vi "HydroCal.vi"() -> ()   [LabVIEW 2022 SP3]
uses:
  ScanningControl/Motion Controllers/NI_controller/-NI_MotionRoutines/MotionSys.ctl
  ScanningControl/Motion Controllers/-MotionRoutines/ScanAxis.ctl
  <vilib>/Math Plots/3D Math Plots/3D Surface/3D Surface XCtrl/3D Surface.xctl
  -CalTransducer/HydrophoneSettings.ctl
  -CalTransducer/Hydros.ctl
  ScanningControl/Digitizers/-DigitizerRoutines/DigitizerSettings.ctl
  ScanningControl/Digitizers/-DigitizerRoutines/Digitizer.ctl
  ScanningControl/Digitizers/-DigitizerRoutines/DigConfig.ctl
  ScanningControl/Digitizers/-DigitizerRoutines/DigitizerID.ctl
  <instrlib>/niSwitch/niSwitch.llb/niSwitch Topologies.ctl
  ScanningControl/Motion Controllers/NI_controller/-NI_MotionRoutines/MotionParameters.ctl
  ScanningControl/Motion Controllers/-MotionRoutines/3rdAxis.ctl
  <vilib>/Analysis/baseanly.llb/Mean (DBL).vi
  <vilib>/Analysis/5stat.llb/RMS (DBL).vi
  ScanningControl/Motion Controllers/-MotionRoutines/MotionGlobals.vi
  <instrlib>/niSwitch/niSwitch.llb/niSwitch Connect Channels (Single).vi
  <vilib>/Math Plots/3D Math Plots/3D Surface/3D Surface Datatype/Public/Plot Helper (Vector).vi
  <instrlib>/niScope/Acquire/Fetch/niScope Multi Fetch.vi
  <vilib>/Utility/file.llb/Write To Spreadsheet File (DBL).vi
  C:/Windows/System32/ADQAPI_dotNet_helper.dll
  <vilib>/Analysis/NI_AALPro.lvlib
  <vilib>/Math Plots/3D Math Plots/3D Surface/3D Surface Datatype/3D Surface Datatype.lvclass
  <vilib>/Analysis/NI_AALBase.lvlib
panel:
  in  "Pressure Cal Parameters":T1={"Center Freq (MHz)"=0.0, "PRF (kHz)"=1.0, "Pulse window (us)"=0.0, "Hydrophone"=enum."PAL #1048", "booster amp?"=TRUE} {"Pulse window (us)" format="%.2f"; "PRF (kHz)" format="%.2f"; "Center Freq (MHz)" format="%.2f"}
  in  "data out":dbl[][][](array[numeric])
  in  "reset mux":bool=TRUE caption="reset mx"
  in  "FileName":string="H"
  in  "Folder":path=path "E:/Temp"
  out "Current Element":i32
  in  "Plot":enum32{"1-D", "2-D", "data", "Spectra"}(tab)
  out "XY Graph":cluster{"axis 1 ticks":dbl[], "data out":dbl[]}(graph)
  in  "Scan":i16=20
  out "3D Surface":refnum<class "3D Plot Datatype.lvclass">[](xcontrol)
  out "Raw Waveforms":dbl[][](graph)
  out "Rms":dbl[](graph)
  out "centers":dbl[][](array[numeric])
  out "Waveform Graph":cluster{i32, "df":dbl, dbl[][]}(graph)
  in  "FFT size":u16(ring) items=["next 2^n", "8", "16", "32", "64", "128", "256", "512", "1024", "2056"]
  in  "home":bool
  in  "Man Cont":bool
  in  "Set up Digi":bool
  in  "Element spacing (mm)":dbl=-1.25
  in  "Elements":i16=20
  in  "scan pair":T3
  in  "Motion System":T4=enum."No Motion Card"
  in  "Motion Bd ID":u8=1 min=1 max=32 step=1
  in  "Location":u16(ring) items=["RRI", "Hawaii", "Cornell", "MM Test"]
  in  "booster amp?":bool=TRUE
  out "Error Message":string
  in  "Type of scan":u16(ring) items=["1-D Scan", "2-D Scan"]
  in  "# of pts per scan":i32=11
  in  "Scan Length (mm)":dbl=5.0 format="%.2f"
  in  "scan":bool
  in  "ExitSendCmd":bool
  # "Use 2.25 unfocused Panametrics at about 65 mm standoff. 25 cycles and 100 mV from Agilent seems good. 600 rf pts seems good and offset to show start of burst. RMS values computed with 400 pts"
  # "Motion Control"
  # "© 2000-2009 WCM"
  # "Note that channels 17-20 have voltage reduced by factor of 1.0476 to account for different cable path lengths. All channels use Miteq amps."
  # "y mm"
  # "z mm"
  # "rms"
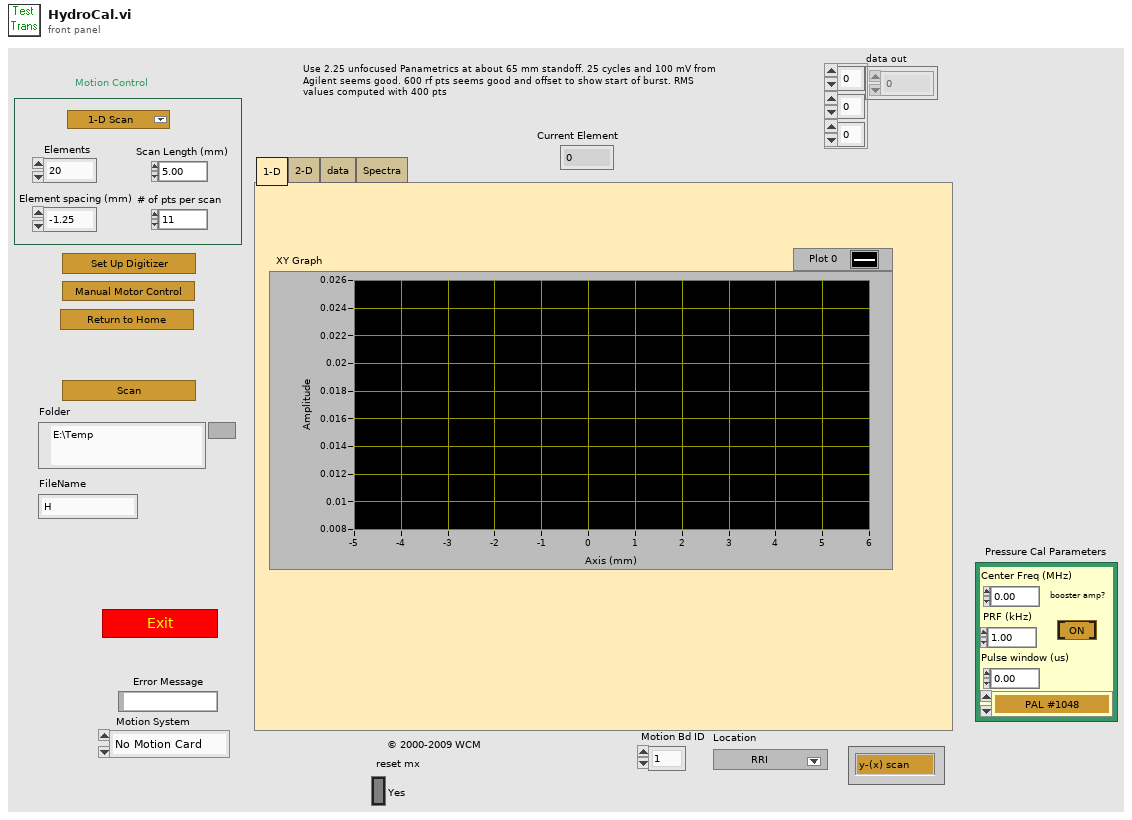
[diagram p1: front panel]
types:
  T1 = typedef "HydrophoneSettings.ctl" = cluster{"Center Freq (MHz)":dbl, "PRF (kHz)":dbl, "Pulse window (us)":dbl, "Hydrophone":T2, "booster amp?":bool}
  T2 = typedef "Hydros.ctl" = enum16{"PAL #1048", "PAL #525", "PAL #430a", "PAL #192", "DEAD PAL # 1403", "LOST UHI Onda", "DEAD PAL #1818", "PAL #1974", "DEAD #2266 w/booster", "PAL #2524 w/booster", "PAL FP21-20T", "PAL FP160-13  ", "PAL FP141-20", "PAL FP158-08T"}
  T3 = typedef "ScanAxis.ctl" = enum16{"y-(x) scan", "x-(y) scan", "z-(x) scan", "z-(y) scan", "y-(z) scan", "x-(z) scan", "w-(x) scan", "w-(y) scan", "w-(z) scan", "x-(w) scan", "y-(w) scan", "z-(w) scan"}
  T4 = typedef "MotionSys.ctl" = enum16{"MM3000", "NI 735x", "Newport ESP", "No Motion Card", "Galil"}
  T5 = typedef "DigitizerSettings.ctl" = cluster{"Digitizer delay (us) ":dbl, "rf points per line":i32, "lines per plane":i32, "Samp Rate (Hz)":dbl, "Additional dig delay (us)":dbl, "Voltage Scale":dbl, "Pre-Looks":i32, "Offset delay (us)":dbl, "bits A/D":i8, "Avg Num":i32, "DigTimeOut":sgl, "Rel Dig Delay":sgl, "Dig Ch":i32, "LeCroyCluster":cluster{"LeCroy Channels":bool[], "LC read pt offset":dbl, "Sweep Avg":bool}, "Main Digitizer":T6, "Dig Config":T7, "Digitizer ID Cluster":T8, "Trigger Settings":cluster{"Trig Source":u16, "Trig Coupling":u16, "Trig Slope":u16, "Level (mV)":dbl}, "Bulk Acq":bool, "Bulk Start Indexes":i32[], "Data Ref RF":refnum<data-value>, "NI ID/Channel":cluster{"NI ID":refnum<k15>, "NI CH":i32}[], "Total Dig CH":i32, "Xtra Ann Trig delay (us)":dbl, "Fix Z Delay?":bool, "One Way Transmission?":bool, "Data Ref Log":refnum<data-value>}
  T6 = typedef "Digitizer.ctl" = enum16{"Acqiris Digitizer", "NI Digitizer", "LeCroy", "GaGe", "AlazarTech", "No Digitizer", "Teledyne"}
  T7 = typedef "DigConfig.ctl" = enum16{"Single channel", "2 Chans w/ 2 Acqiris", "2 Chans w/ 1 Acqiris", "5-CH Pulser New", "5-CH pulser w/ ann array", "5-pass style ann array", "Empty"}
  T8 = typedef "DigitizerID.ctl" = cluster{"Acqiris/Alazar/SP ID":u32[], "NI Instr Handles":refnum<k15>[], "LeCroy VISA":refnum<visa-resource-name>, "GaGe Handle":cluster{"Handle":u32, "Sample size":u32, "Resolution":i32, "Offset":i32, "Channels":u32, "Boards":u32}, "ATS Ref":string, "Acqiris Address":string[], "ADQRef":refnum<k24>, "adq_cu_ptr":refnum<k24>}
  T9 = typedef "niSwitch Topologies.ctl" = string
  T10 = enum16{"Absolute Position", "Relative Position", "Velocity", "Relative to Cap Pos", "Modulus Position", "Absolute Contouring", "Relative Contouring"}
  T11 = typedef "MotionParameters.ctl" = cluster{"No Motion?":bool, "Motion System":T4, "Motion Bd ID":u8, "Motion Profile":string, "# Axis":i8, "Reverse Z axis?":bool, "SMAC Axis":u16, "scan pair":T3, "RT fps":sgl, "Steps per mm":i32[], "Motor Parameters":cluster{"velocity ct/s":dbl[], "accel ct/s^2":dbl[]}, "One Way Scan":bool, "Reverse One Way Scan":bool, "Global Position (mm)":dbl[], "Plane":i32, "Distance between\nscan lines (um)":sgl, "Distance between\nscan planes (um)":sgl, "number of scan planes":i32, "Total steps in line":i32, "Xtra plane\ndistance  (um)":i32, "Xtra planes ":i32, "Add Axis":bool, "overshoot cts":i32, "BKPT Shift":i32, "Scan Start Time (ms)":u32, "ESP VISA":refnum<visa-resource-name>, "3rd Axis":T12, "GL Ref Out":refnum<k7>, "Galil Address":string}
  T12 = typedef "3rdAxis.ctl" = u16
  T13 = cluster{"scan data":dbl[][][], "Pulse Parameters":cluster{"Frequency (MHz)":dbl, "prf":dbl, "focal length (cm)":dbl, "derating (.3) factor":dbl, "neg peak pressure (MPa)":dbl, "pos peak pressure (MPa)":dbl, "p.3":dbl, "pulse dur (Pd s)":dbl, "Pulse Int \nIntegral (PII J/cm^2)":dbl, "Pulse Av Intensity\n (Ipa W/cm^2)":dbl, "Ipa.3":dbl, "Temporal Av Intensity \n(Ita mW/cm^2)":dbl, "Ita.3":dbl, "MI":dbl}[][], "axis1o":dbl, "axis2o":dbl, "step size":dbl, "axis 1 ticks":dbl[], "axis 2 ticks":dbl[]}
  T14 = cluster{"actualSamples":i32, "absoluteInitialX":dbl, "relativeInitialX":dbl, "xIncrement":dbl, "offset":dbl, "gain":dbl, "reserved1":dbl, "reserved2":dbl}[]
  T15 = cluster{"actualSamples":i32, "absoluteInitialX":dbl, "relativeInitialX":dbl, "xIncrement":dbl, "offset":dbl, "gain":dbl, "reserved1":dbl, "reserved2":dbl}
  T16 = typedef "AnnularArray.ctl" = cluster{"Synth Foc?":bool, "Focal Zones":i16, "Switch T/R":i16, "Trans Geometry (mm)":T17, "Sub Ap Excite?":bool, "Full Array Scan?":bool, "Xmt/Rcv":cluster{"XMIT":bool[], "RCV":bool[]}, "PulseSpacing (us)":sgl, "Xmit Ring":i32, "XMIT CHS":u8, "RCV CHS":u8, "GPU?":bool, "Save TIFF?":bool, "downfactor":i32, "RCV 1CH":u16}
  T17 = typedef "TransGeometry.ctl" = cluster{"Transducer":T18, "Geo Focus":dbl, "a (radius)":dbl, "# of rings":i32, "kerf space ":dbl, "Center Freq":dbl}
  T18 = typedef "ArrayGeometry.ctl" = u16
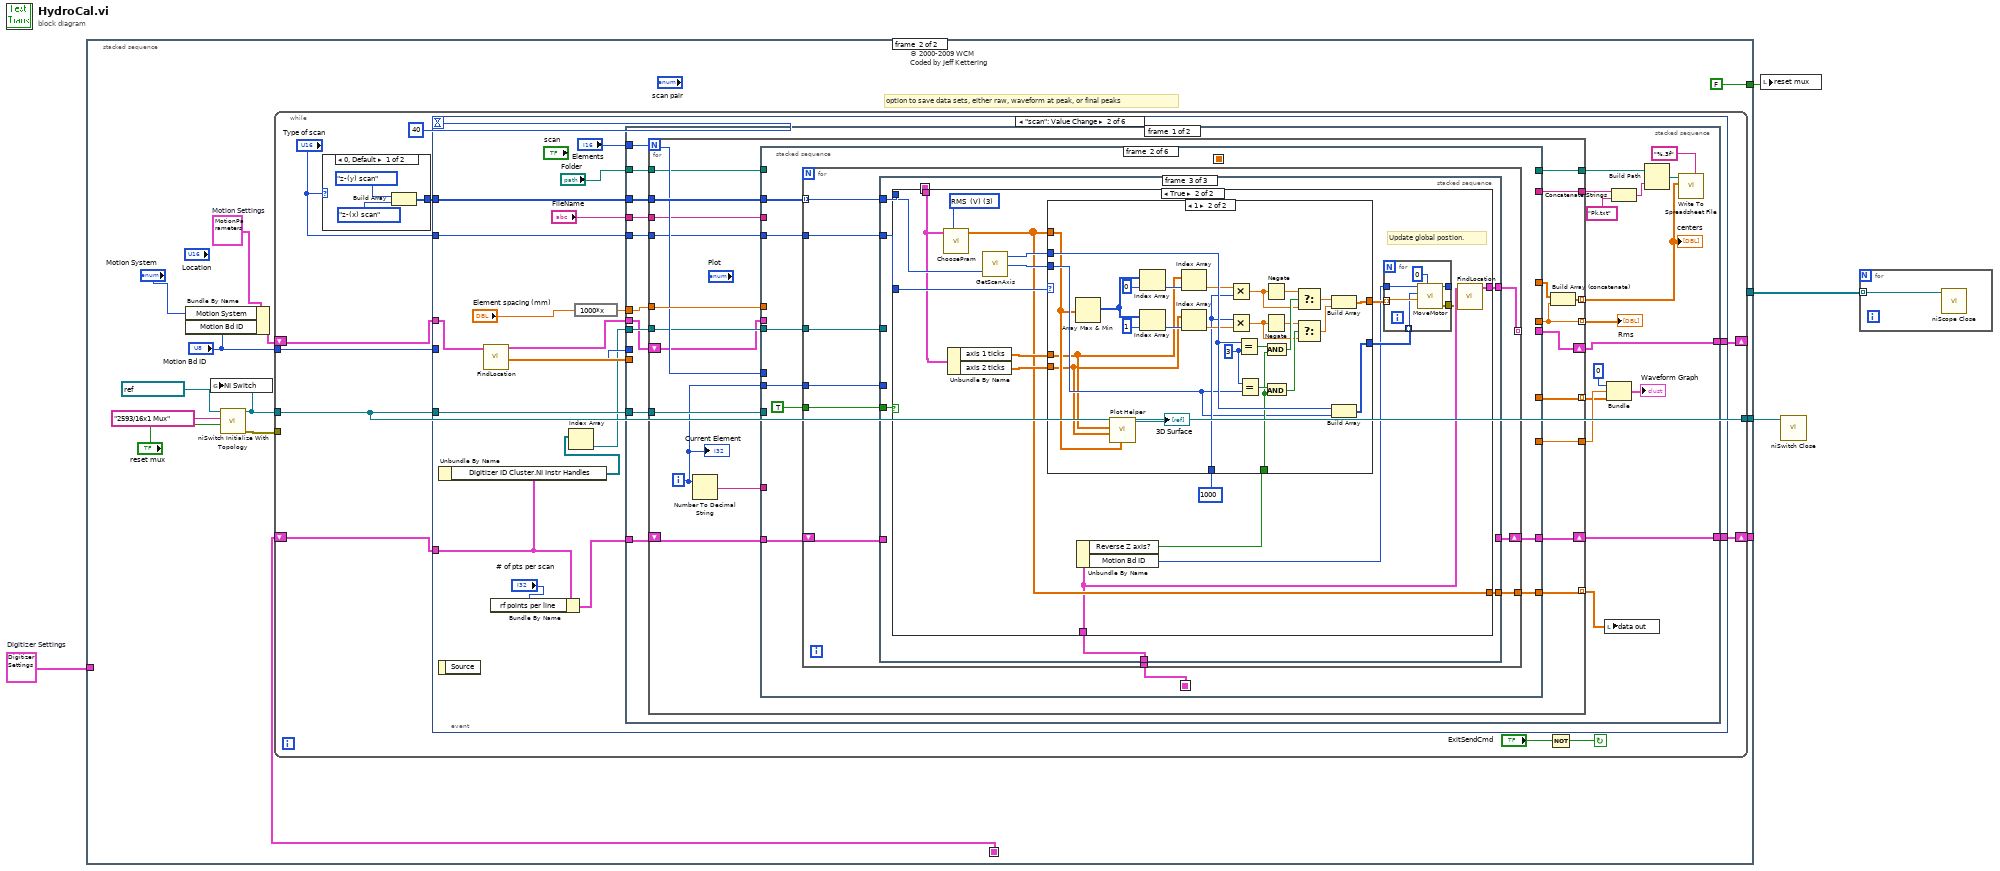
[diagram p0: block diagram]
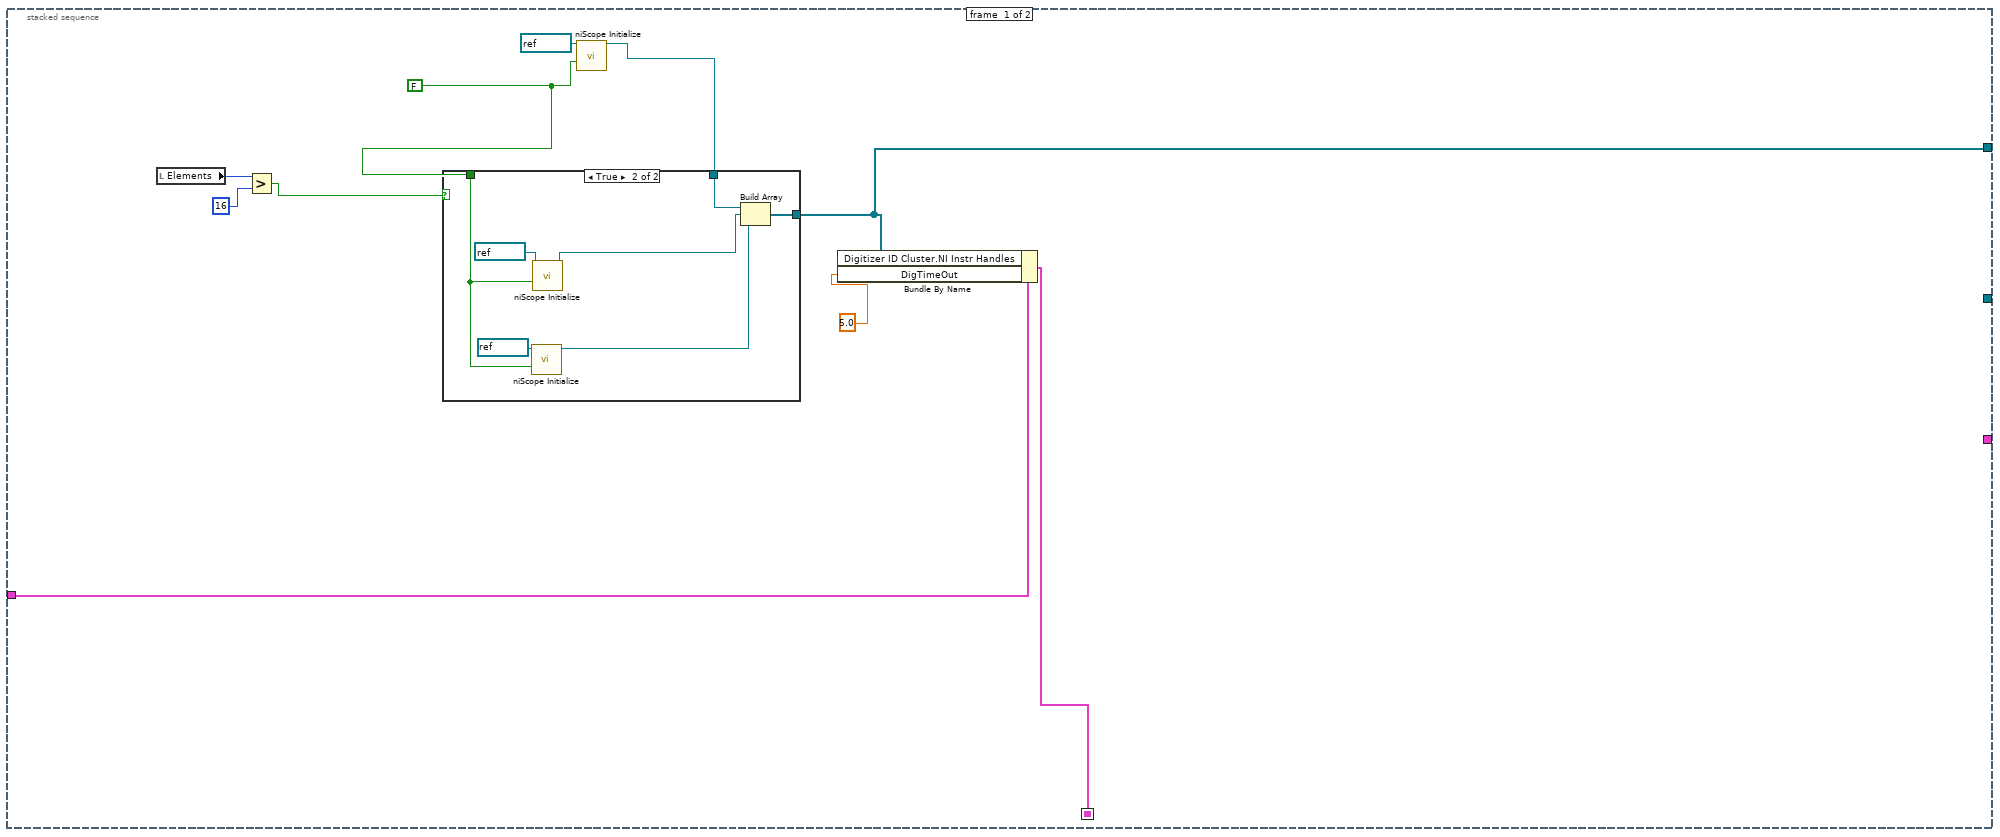
[diagram p2: hidden frame]
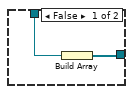
[diagram p3: hidden frame]
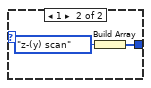
[diagram p4: hidden frame]
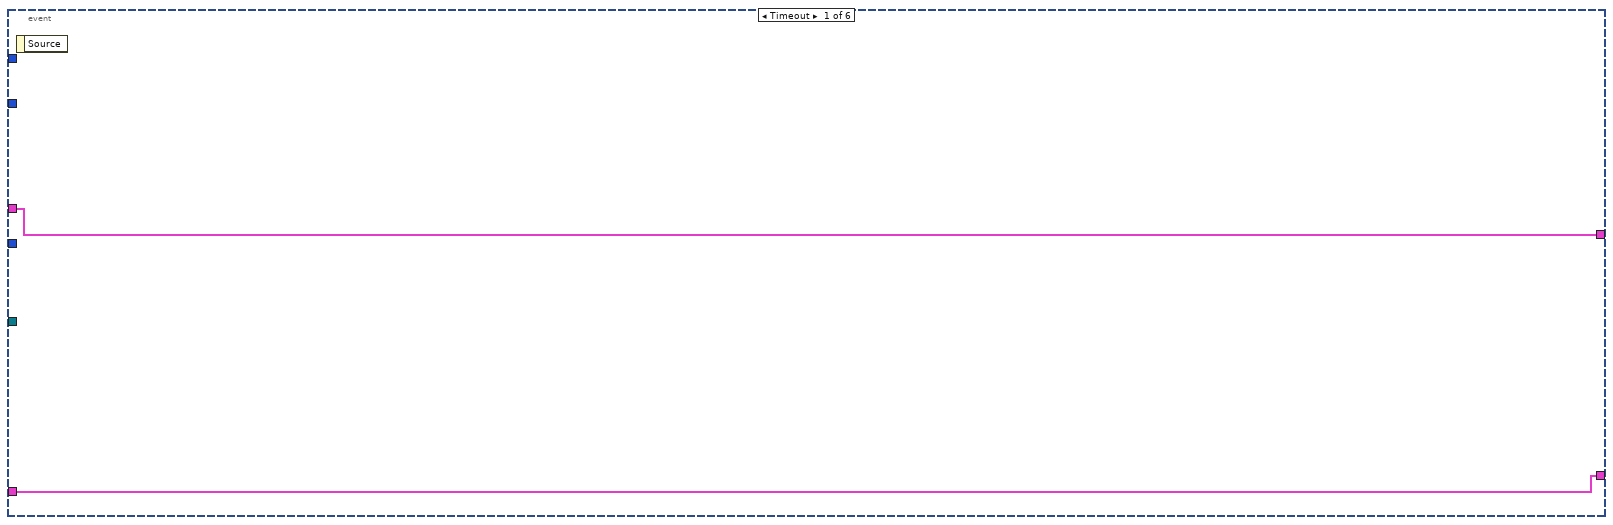
[diagram p5: hidden frame]
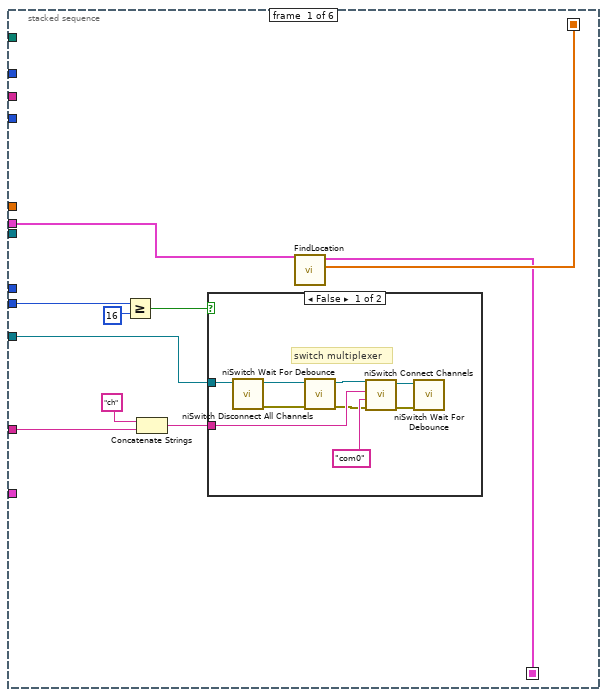
[diagram p6: hidden frame]
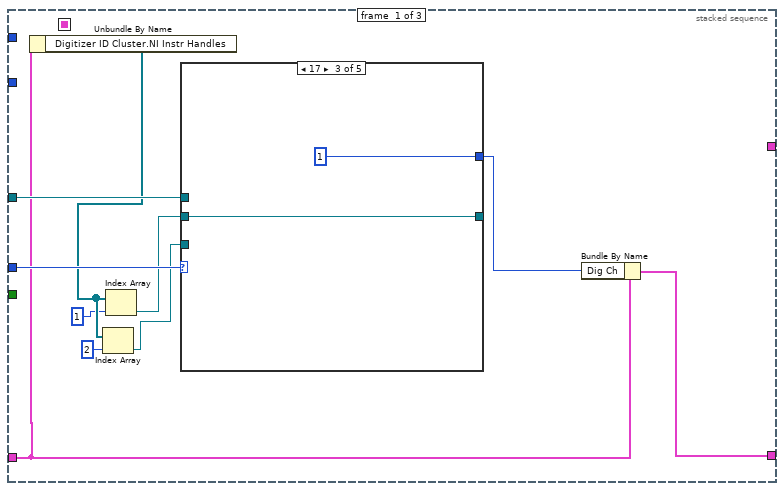
[diagram p8: hidden frame]
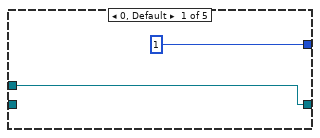
[diagram p9: hidden frame]
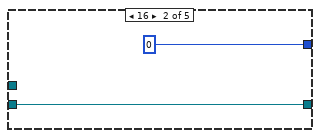
[diagram p10: hidden frame]
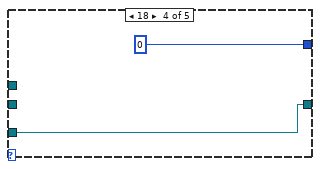
[diagram p11: hidden frame]
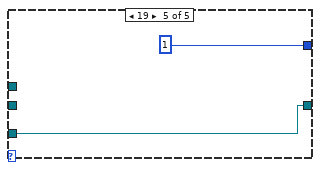
[diagram p12: hidden frame]
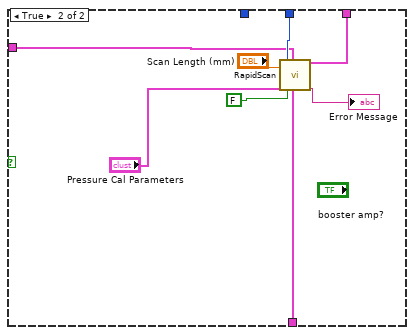
[diagram p14: hidden frame]
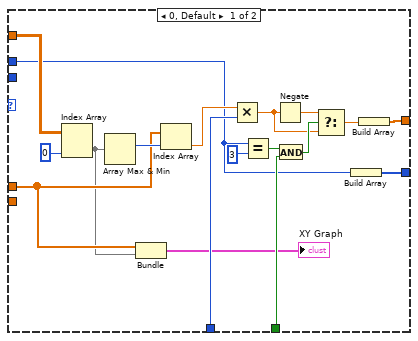
[diagram p16: hidden frame]
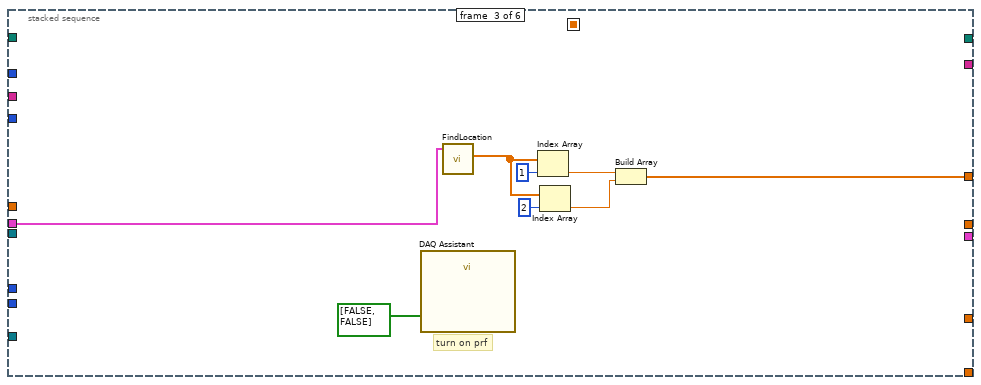
[diagram p17: hidden frame]
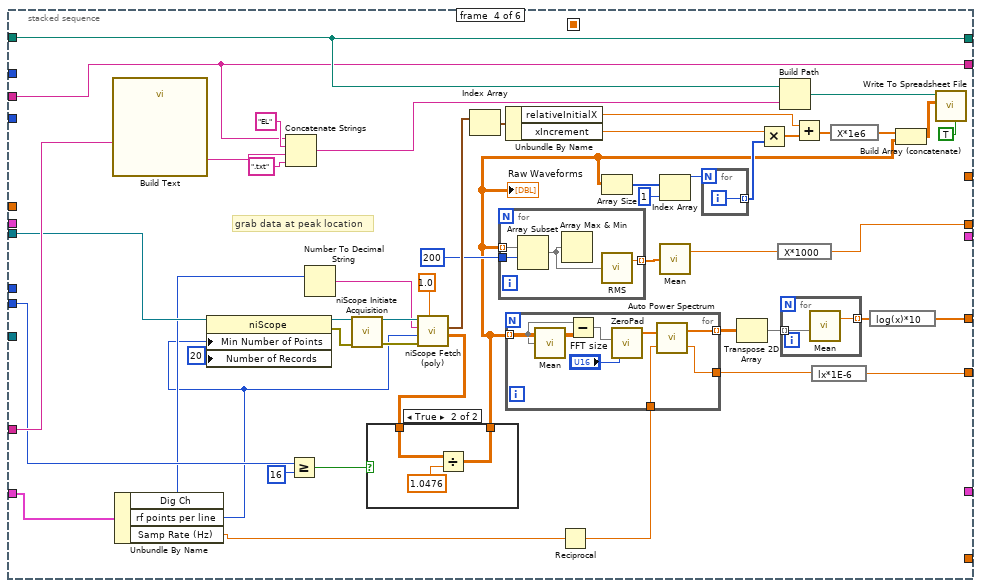
[diagram p18: hidden frame]
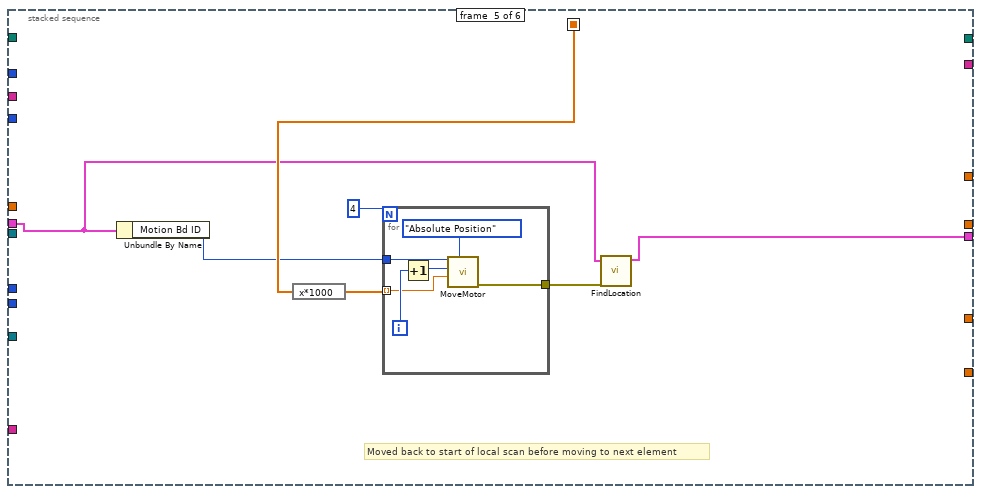
[diagram p20: hidden frame]
diagram:
  w1 = T5 {"Digitizer delay (us) "=0.0, "rf points per line"=2048, "lines per plane"=128, "Samp Rate (Hz)"=100000000.0, "Additional dig delay (us)"=0.0, "Voltage Scale"=0.4, "Pre-Looks"=0, "Offset delay (us)"=0.0, "bits A/D"=8, "Avg Num"=1, "DigTimeOut"=5.0, "Rel Dig Delay"=0.0, "Dig Ch"=0, "LeCroyCluster"={"LeCroy Channels"=[TRUE, FALSE, FALSE, FALSE], "LC read pt offset"=0.0, "Sweep Avg"=FALSE}, "Main Digitizer"=enum."NI Digitizer", "Dig Config"=enum."Single channel", "Digitizer ID Cluster"={"Acqiris/Alazar/SP ID"=[], "NI Instr Handles"=[], "LeCroy VISA"="", "GaGe Handle"={"Handle"=0, "Sample size"=0, "Resolution"=0, "Offset"=0, "Channels"=0, "Boards"=0}, "ATS Ref"="ATS9350", "Acqiris Address"=["PCI::INSTR0"], "ADQRef"=refnum, "adq_cu_ptr"=refnum}, "Trigger Settings"={"Trig Source"=1, "Trig Coupling"=0, "Trig Slope"=0, "Level (mV)"=1500.0}, "Bulk Acq"=FALSE, "Bulk Start Indexes"=[], "Data Ref RF"=refnum, "NI ID/Channel"=[], "Total Dig CH"=5, "Xtra Ann Trig delay (us)"=10.0, "Fix Z Delay?"=FALSE, "One Way Transmission?"=FALSE, "Data Ref Log"=refnum}  # Digitizer Settings
  n1 = stacked-sequence {
    seq-local: [w5 _] -> [_ w29]
    tunnel: [_ w34] -> w4
    tunnel: [_ FALSE ("reset device (boolean value)")] -> w3
    tunnel: [w8 _] -> w2
    tunnel: w1 -> [w7 _]
    tunnel: [_ w24] -> _
    frame #0 {
      w10 = FALSE
      n2 = local read "Elements"() -> (w13:i16)
      n3 = Greater?(x=w13, y=16) -> (0:w11:bool)
      n4 = call <instrlib>:"niScope Initialize.vi"("resource name"=refnum<k15> "DIG1", "reset device"=w10) -> ("instrument handle"=w9:refnum<k15>)  [unwired: 2 in, 11 out]
      n5 = case shown="True" w11 {
        tunnel: w10 -> [_ w21]
        tunnel: w9 -> [w16 w20]
        tunnel: [w15 w17] -> w8
        frame False {
          n6 = Build Array(w16) -> (w15:refnum<k15>[])
        }
        frame True {
          n7 = call <instrlib>:"niScope Initialize.vi"("resource name"=refnum<k15> "DIG3", "reset device"=w21) -> ("instrument handle"=w18:refnum<k15>)  [unwired: 2 in, 11 out]
          n8 = call <instrlib>:"niScope Initialize.vi"("resource name"=refnum<k15> "DIG2", "reset device"=w21) -> ("instrument handle"=w19:refnum<k15>)  [unwired: 2 in, 11 out]
          n9 = Build Array(w20, w19, w18) -> (w17:refnum<k15>[])
        }
      }
      n10 = Bundle By Name(cluster=w7, "Digitizer ID Cluster.NI Instr Handles"=w8, "DigTimeOut"=sgl 5.0) -> (w5:T5)
    }
    frame #1 {
      w26 = T11 {"No Motion?"=FALSE, "Motion System"=enum."No Motion Card", "Motion Bd ID"=1, "Motion Profile"="SMAC1", "# Axis"=1, "Reverse Z axis?"=TRUE, "SMAC Axis"=0, "scan pair"=enum."y-(x) scan", "RT fps"=6.0, "Steps per mm"=[1000, 1000, 1000, 1000], "Motor Parameters"={"velocity ct/s"=[10000.0, 10000.0, 10000.0, 50000.0], "accel ct/s^2"=[50000.0, 50000.0, 50000.0, 200000.0]}, "One Way Scan"=FALSE, "Reverse One Way Scan"=FALSE, "Global Position (mm)"=[], "Plane"=0, "Distance between\nscan lines (um)"=0.0, "Distance between\nscan planes (um)"=0.0, "number of scan planes"=1, "Total steps in line"=0, "Xtra plane\ndistance  (um)"=100, "Xtra planes "=1, "Add Axis"=FALSE, "overshoot cts"=200, "BKPT Shift"=0, "Scan Start Time (ms)"=0, "ESP VISA"="GPIB::1::INSTR", "3rd Axis"=1, "GL Ref Out"=refnum, "Galil Address"=""}  # Motion Settings
      # "option to save data sets, either raw, waveform at peak, or final peaks"
      # "© 2000-2009 WCM\nCoded by Jeff Kettering"
      n11 = Bundle By Name(cluster=w26, "Motion System"="Motion System", "Motion Bd ID"="Motion Bd ID") -> (w25:T11)
      n12 = call <instrlib>:"niSwitch Initialize With Topology.vi"("reset device (boolean value)"="reset mux", "topology name"=T9 "2593/16x1 Mux", "resource name"=refnum<k15> "PXI1Slot5") -> ("error out"=w35:errorcluster, "instrument handle out"=w32:refnum<k15>)  [unwired: 7 in]
      n13 = global write "MotionGlobals.vi" "NI Switch"(w32) -> ()
      n14 = while {
        tunnel: "Motion Bd ID" -> [w44]
        tunnel: w32 -> [w42]
        tunnel: w35 -> [_]
        tunnel: [w42] -> w34
        shift-right: [w38] -> w24
        shift-left: w29 -> [w40]
        shift-right: [w37] -> _
        shift-left: w25 -> [w39]
        stop <- w46 continue-if-true
        n15 = case shown="0, Default" "Type of scan" {
          tunnel: [w48 w52] -> w43
          frame 0, Default {
            n16 = Build Array(ScanAxis."z-(y) scan" ("scan pair"), ScanAxis."z-(x) scan" ("scan pair")) -> (w48:T3[])
          }
          frame 1 {
            n17 = Build Array(ScanAxis."z-(y) scan" ("scan pair")) -> (w52:T3[])
          }
        }
        n18 = event shown="[1] \"scan\": Value Change" {
          selector: _ -> [_ _ _ _ _ _]
          dyn-events: _ -> [_ _ _ _ _ _]
          timeout: 40 -> [_ _ _ _ _ _]
          tunnel: w44 -> [_ _ _ _ w428 _]
          tunnel: w42 -> [_ w72 w403 _ _ _]
          tunnel: w43 -> [_ w71 _ _ _ _]
          tunnel: "Type of scan" -> [_ w68 _ _ _ _]
          tunnel: w40 -> [w53 w57 w402 w417 w427 w429]
          tunnel: w39 -> [w54 w61 w400 w416 w425 w430]
          tunnel: [w53 w59 w401 w417 w427 w429] -> w38
          tunnel: [w54 w55 w399 w415 w424 w430] -> w37
          event Timeout {
            n19 = event-data() -> ()  [unwired: 2 out]
          }
          event "scan": Value Change {
            n20 = Unbundle By Name(w57) -> ("Digitizer ID Cluster.NI Instr Handles"=w63:refnum<k15>[])
            n21 = event-data() -> ()  [unwired: 2 out]
            n22 = call "FindLocation.vi"("Motion Settings"=w61) -> ("Motion Settings Out"=w60:T11, "location (mm)"=w67:dbl[], "Bd ID Out"=w66:u8)  [unwired: 2 in, 1 out]
            n23 = Bundle By Name(cluster=w57, "rf points per line"="# of pts per scan") -> (w56:T5)
            n24 = Index Array(array=w63) -> (element=w62:refnum<k15>)  [unwired: 1 in]
            n25 = expression code="1000*x"("Element spacing (mm)") -> (w69:dbl)
            n26 = stacked-sequence {
              tunnel: w66 -> [_ w379]
              tunnel: "Elements" -> [w98 _]
              tunnel: w72 -> [w97 w384]
              tunnel: w71 -> [w96 _]
              tunnel: w69 -> [w95 _]
              tunnel: w68 -> [w94 _]
              tunnel: w67 -> [_ w380]
              tunnel: "Folder" -> [w87 _]
              tunnel: "FileName" -> [w86 _]
              tunnel: w62 -> [w85 _]
              tunnel: w56 -> [w77 w376]
              tunnel: w60 -> [w76 w377]
              tunnel: [w75 _] -> w59
              tunnel: [w74 _] -> w55
              frame #0 {
                n27 = for {
                  N: w98 -> [w116]
                  tunnel: w97 -> [w120]
                  tunnel: w96 -> [w118]
                  tunnel: w95 -> [w117]
                  tunnel: [w105] -> w93 mode=indexing
                  tunnel: [w114] -> w82 mode=indexing
                  tunnel: w94 -> [w113]
                  tunnel: [w112] -> w91
                  tunnel: [w111] -> w90
                  tunnel: w87 -> [w110]
                  tunnel: w86 -> [w109]
                  tunnel: w85 -> [w108]
                  tunnel: [w107] -> w84
                  tunnel: [w104] -> w79 mode=indexing
                  tunnel: [w103] -> w78 mode=indexing
                  shift-right: [w100] -> w75
                  shift-left: w77 -> [w102]
                  shift-right: [w99] -> w74
                  shift-left: w76 -> [w101]
                  i -> [w115]
                  n28 = Number To Decimal String(number=w115) -> (decimal integer string=w119:string)  [unwired: 1 in]
                  n29 = stacked-sequence {
                    seq-local: [w126 _ _ _ _ _] -> [_ _ _ _ w350 _]
                    seq-local: [w121 _ _ _ _ _] -> [_ w140 _ _ _ _]
                    tunnel: w118 -> [_ w148 _ _ _ w364]
                    tunnel: w120 -> [w127 _ _ _ _ _]
                    tunnel: w119 -> [w130 _ _ w316 _ _]
                    tunnel: w117 -> [_ _ _ _ _ w365]
                    tunnel: [_ _ w272 _ _ _] -> w106
                    tunnel: w116 -> [_ _ _ _ _ w362]
                    tunnel: w115 -> [w125 w145 _ w285 _ w361]
                    tunnel: [_ _ _ w288 _ _] -> w105
                    tunnel: [_ _ _ w317 _ _] -> w114
                    tunnel: w113 -> [_ w147 _ _ _ _]
                    tunnel: [_ _ _ w309 _ _] -> w112
                    tunnel: [_ _ _ w310 _ _] -> w111
                    tunnel: w110 -> [_ _ _ w310 _ _]
                    tunnel: w109 -> [_ _ _ w309 _ _]
                    tunnel: w108 -> [_ w146 _ w282 _ _]
                    tunnel: [_ _ _ w291 _ _] -> w107
                    tunnel: [_ w144 _ _ _ _] -> w103
                    tunnel: w102 -> [_ w142 _ w281 _ _]
                    tunnel: w101 -> [w122 _ w270 _ w348 w359]
                    tunnel: [_ w141 _ _ _ _] -> w100
                    tunnel: [_ _ _ _ w346 _] -> w99
                    frame #0 {
                      n30 = Greater Or Equal?(x=w125, y=16) -> (x >= y?=w123:bool)
                      n31 = Concatenate Strings("ch", w130) -> (w128:string)
                      n32 = case shown="False" w123 {
                        tunnel: w128 -> [w139 _]
                        tunnel: w127 -> [w135 _]
                        frame False {
                          # "switch multiplexer"
                          n33 = call <instrlib>:"niSwitch Disconnect All Channels.vi"("instrument handle"=w135) -> ("error out"=w131:errorcluster, "instrument handle out"=w134:refnum<k15>)  [unwired: 9 in]
                          n34 = call <instrlib>:"niSwitch Wait For Debounce.vi"("error in (no error)"=w131, "instrument handle"=w134) -> ("error out"=w132:errorcluster, "instrument handle out"=w133:refnum<k15>)  [unwired: 8 in]
                          n35 = call-poly <instrlib>:"niSwitch Connect Channels.vi"("error in (no error)"=w132, "channel 2"="com0", "channel 1"=w139, "instrument handle"=w133) -> ("error out"=w137:errorcluster, "instrument handle out"=w136:refnum<k15>)  [unwired: 6 in]
                          n36 = call <instrlib>:"niSwitch Wait For Debounce.vi"("error in (no error)"=w137, "instrument handle"=w136) -> ()  [unwired: 8 in, 2 out]
                        }
                        frame True {
                        }
                      }
                      n37 = call "FindLocation.vi"("Motion Settings"=w122) -> ("Motion Settings Out"=w121:T11, "location (mm)"=w126:dbl[])  [unwired: 2 in, 2 out]
                    }
                    frame #1 {
                      n38 = for {
                        tunnel: w148 -> [w158] mode=indexing
                        tunnel: w147 -> [w157]
                        tunnel: w146 -> [w156]
                        tunnel: w145 -> [w155]
                        tunnel: [w154] -> w144
                        tunnel: TRUE -> [w153]
                        shift-right: [w151] -> w141
                        shift-left: w142 -> [w152]
                        tunnel: w140 -> [w150]
                        tunnel: [w149] -> _ mode=indexing
                        n39 = stacked-sequence {
                          seq-local: [_ w183 _] -> [_ _ w197]
                          tunnel: w158 -> [_ w184 w199]
                          tunnel: w157 -> [_ w182 w198]
                          tunnel: w155 -> [w168 _ _]
                          tunnel: w156 -> [w167 _ _]
                          tunnel: [_ _ w196] -> w154
                          tunnel: w153 -> [_ w181 w195]
                          tunnel: w152 -> [w161 w180 _]
                          tunnel: [w159 _ _] -> w151
                          tunnel: w150 -> [_ w179 w194]
                          tunnel: [_ _ w193] -> w149
                          frame #0 {
                            n40 = Unbundle By Name(w161) -> ("Digitizer ID Cluster.NI Instr Handles"=w165:refnum<k15>[])
                            n41 = Index Array(array=w165, index=2) -> (element=w163:refnum<k15>)
                            n42 = Index Array(array=w165, index=1) -> (element=w164:refnum<k15>)
                            n43 = case shown="17" w168 {
                              tunnel: w164 -> [_ w172 w174 _ _]
                              tunnel: [w170 w172 w174 w176 w178] -> _
                              tunnel: w163 -> [_ _ _ w176 w178]
                              tunnel: w167 -> [w170 _ _ _ _]
                              tunnel: [1 0 1 0 1] -> w160
                              frame 0, Default {
                              }
                              frame 16 {
                              }
                              frame 17 {
                              }
                              frame 18 {
                              }
                              frame 19 {
                              }
                            }
                            n44 = Bundle By Name(cluster=w161, "Dig Ch"=w160) -> (w159:T5)
                          }
                          frame #1 {
                            n45 = case shown="False" w181 {
                              tunnel: w184 -> [_ _]
                              tunnel: [_ w189] -> w183
                              tunnel: w182 -> [_ w188]
                              tunnel: w180 -> [_ w186]
                              tunnel: w179 -> [_ w187]
                              frame False {
                              }
                              frame True {
                                n46 = call "RapidScan.vi"("Scan Length (mm)"="Scan Length (mm)", "Pressure Cal Parameters"="Pressure Cal Parameters", "Type of scan"=w188, "Therapy"=FALSE, "Digitizer Settings"=w186, "Motion Settings"=w187) -> ("Scan data"=w189:T13, "Error Message"=→"Error Message":string)  [unwired: 9 in, 3 out]
                              }
                            }
                          }
                          frame #2 {
                            n47 = case shown="True" w195 {
                              tunnel: w199 -> [_ w217]
                              tunnel: w198 -> [_ w209]
                              tunnel: w197 -> [_ w207]
                              tunnel: [_ w206] -> w196
                              tunnel: w194 -> [w200 w203]
                              tunnel: [w200 w201] -> w193
                              frame False {
                              }
                              frame True {
                                w208 = u16 3 items=["Neg Peak (V)", "Pos Peak  (V)", "Peak to Peak  (V)", "RMS  (V)", "Neg Peak Pressure (MPa)", "p.3 (MPa)", "Ipa (W/cm^2)", "Ipa.3 (W/cm^2)", "Ita (W/cm^2)", "Ita.3 (W/cm^2)"] ("Parameter Selection")
                                # "Update global postion."
                                n48 = call "ChoosePram.vi"("Parameter Selection"=w208, "Scan data"=w207) -> ("data out"=w206:dbl[][])  [unwired: 2 in, 7 out]
                                n49 = Unbundle By Name(w207) -> ("axis 1 ticks"=w216:dbl[], "axis 2 ticks"=w215:dbl[])
                                n50 = call "GetScanAxis.vi"("scan pair"=w217) -> ("Axis 1"=w211:i32, "Axis 2"=w210:i32)  [unwired: 1 in, 1 out]
                                n51 = Unbundle By Name(w203) -> ("Reverse Z axis?"=w204:bool, "Motion Bd ID"=w205:u8)
                                n52 = case shown="1" w209 {
                                tunnel: w206 -> [w235 w238]
                                tunnel: w204 -> [w234 w242]
                                tunnel: [w233 w260] -> w213
                                tunnel: [w232 w259] -> w214
                                tunnel: w211 -> [w221 w257]
                                tunnel: w210 -> [_ w240]
                                tunnel: w216 -> [w220 w237]
                                tunnel: 1000 -> [w231 w244]
                                tunnel: w215 -> [_ w236]
                                frame 0, Default {
                                n53 = Index Array(array=w235, index (col)=0) -> (element=w219:dbl[])  [unwired: 1 in]
                                n54 = Array Max & Min(array=w219) -> (max index (indices)=w224:i32)  [unwired: 3 out]
                                n55 = Bundle("axis 1 ticks"=w220, "data out"=w219) -> (→"XY Graph":cluster{"axis 1 ticks":dbl[], "data out":dbl[]})  [unwired: 1 in]
                                n56 = Index Array(array=w220, index=w224) -> (element=w223:dbl)
                                n57 = Multiply(x=w223, y=w231) -> (x*y=w222:dbl)
                                n58 = Equal?(x=w221, y=3) -> (x = y?=w227:bool)
                                n59 = Negate(x=w222) -> (-x=w229:dbl)
                                n60 = And(x=w227, y=w234) -> (x .and. y?=w226:bool)
                                n61 = Select(t=w229, s=w226, f=w222) -> (s? t:f=w225:dbl)
                                n62 = Build Array(w221) -> (w233:i32[])
                                n63 = Build Array(w225) -> (w232:dbl[])
                                }
                                frame 1 {
                                w241 = 3
                                n64 = Array Max & Min(array=w238) -> (max index (indices)=w250:i32[])  [unwired: 3 out]
                                n65 = call-poly <vilib>:"Plot Helper.vi"("z matrix"=w238, "y vector"=w236, "x vector"=w237) -> ("3D Plot lvclass Array out"=→"3D Surface":refnum<class "3D Plot Datatype.lvclass">[])  [unwired: 3 in, 5 out]
                                n66 = Index Array(array=w250, index=0 ("Index")) -> (element=w249:i32)
                                n67 = Index Array(array=w250, index=1 ("Index")) -> (element=w248:i32)
                                n68 = Index Array(array=w237, index=w249) -> (element=w247:dbl)
                                n69 = Index Array(array=w236, index=w248) -> (element=w245:dbl)
                                n70 = Multiply(x=w247, y=w244) -> (x*y=w246:dbl)
                                n71 = Multiply(x=w244, y=w245) -> (x*y=w243:dbl)
                                n72 = Equal?(x=w257, y=w241) -> (x = y?=w256:bool)
                                n73 = Equal?(x=w241, y=w240) -> (x = y?=w253:bool)
                                n74 = Negate(x=w246) -> (-x=w258:dbl)
                                n75 = Negate(x=w243) -> (-x=w252:dbl)
                                n76 = And(x=w256, y=w242) -> (x .and. y?=w255:bool)
                                n77 = And(x=w253, y=w242) -> (x .and. y?=w254:bool)
                                n78 = Select(t=w258, s=w255, f=w246) -> (s? t:f=w261:dbl)
                                n79 = Select(t=w252, s=w254, f=w243) -> (s? t:f=w251:dbl)
                                n80 = Build Array(w261, w251) -> (w259:dbl[])
                                n81 = Build Array(w257, w240) -> (w260:i32[])
                                }
                                }
                                n82 = for {
                                tunnel: [w269] -> _
                                tunnel: w214 -> [w267] mode=indexing
                                tunnel: w205 -> [w266]
                                tunnel: w213 -> [w265] mode=indexing
                                tunnel: [w264] -> w202
                                n83 = call "MoveMotor.vi"("Position Mode (Absolute)"=0, "Target Position (0)"=w267, "Axis or Vector Space"=w265, "Motion Bd ID"=w266) -> ("error out"=w264:errorcluster, "Bd ID Out"=w269:u8)  [unwired: 1 in, 5 out]
                                }
                                n84 = call "FindLocation.vi"("Motion Settings"=w203, "error in (no error)"=w202) -> ("Motion Settings Out"=w201:T11)  [unwired: 1 in, 3 out]
                              }
                            }
                          }
                        }
                      }
                    }
                    frame #2 {
                      # "turn on prf"
                      n85 = call "DAQ Assistant"("data"=bool[] [FALSE, FALSE]) -> ()  [unwired: 3 in, 16 out]
                      n86 = call "FindLocation.vi"("Motion Settings"=w270) -> ("location (mm)"=w276:dbl[])  [unwired: 2 in, 3 out]
                      n87 = Index Array(array=w276, index=1) -> (element=w274:dbl)
                      n88 = Index Array(array=w276, index=2) -> (element=w273:dbl)
                      n89 = Build Array(w274, w273) -> (w272:dbl[])
                    }
                    frame #3 {
                      # "grab data at peak location"
                      n90 = call "Build Text"("d"=w316) -> ("Result"=w315:string)  [unwired: 13 in, 1 out]
                      n91 = Unbundle By Name(w281) -> ("Dig Ch"=w279:i32, "rf points per line"=w278:i32, "Samp Rate (Hz)"=w280:dbl)
                      n92 = property class="niScope"(reference=w282, "Min Number of Points"=w278, "Number of Records"=20) -> (reference out=w326:refnum<k15>, error out=w325:errorcluster)  [unwired: 1 in]
                      n93 = Concatenate Strings(w309, "EL" ("string"), w315, ".txt") -> (w313:string)
                      n94 = Greater Or Equal?(x=w285, y=16) -> (x >= y?=w284:bool)
                      n95 = Number To Decimal String(number=w279) -> (decimal integer string=w294:string)  [unwired: 1 in]
                      n96 = call <instrlib>:"niScope Initiate Acquisition.vi"("instrument handle"=w326, "error in"=w325) -> ("instrument handle out"=w324:refnum<k15>, "error out"=w323:errorcluster)  [unwired: 12 in]
                      n97 = call-poly <instrlib>:"niScope Fetch (poly).vi"("timeout"=1.0, "error in"=w323, "numSamples"=w278, "channels"=w294, "instrument handle"=w324) -> ("wfm"=w283:dbl[][], "wfm info"=w308:T14)  [unwired: 3 in, 2 out]
                      n98 = case shown="True" w284 {
                        tunnel: w283 -> [w327 w329]
                        tunnel: [w327 w328] -> w287
                        frame False {
                        }
                        frame True {
                          n99 = Divide(x=w329, y=1.0476) -> (x/y=w328:dbl[][])
                        }
                      }
                      "Raw Waveforms" <- w287
                      n100 = Index Array(array=w308) -> (element=w307:T15)  [unwired: 1 in]
                      n101 = for {
                        tunnel: w287 -> [w334] mode=indexing
                        tunnel: [w335] -> w293 mode=indexing
                        tunnel: 200 ("index") -> [w332]
                        n102 = Array Subset(array=w334, index=w332) -> (w333:dbl[])  [unwired: 1 in]
                        n103 = Array Max & Min(array=w333) -> ()  [unwired: 4 out]
                        n104 = call-poly <vilib>:"RMS.vi"("X"=w333) -> ("rms value"=w335:dbl)  [unwired: 1 out]
                      }
                      n105 = Unbundle By Name(w307) -> ("relativeInitialX"=w300:dbl, "xIncrement"=w302:dbl)
                      n106 = Reciprocal(x=w280) -> (1/x=w321:dbl)
                      n107 = for {
                        tunnel: w287 -> [w344] mode=indexing
                        tunnel: [w343] -> w319 mode=indexing
                        tunnel: w321 -> [w342]
                        tunnel: [w341] -> w292
                        n108 = call-poly <vilib>:"Mean.vi"("X"=w344) -> ("mean"=w345:dbl)  [unwired: 1 out]
                        n109 = Subtract(x=w344, y=w345) -> (x-y=w340:dbl[])
                        n110 = call "ZeroPad.vi"("Input Array"=w340, "FFT size"="FFT size") -> ("Ouput Array"=w339:dbl[])  [unwired: 3 in, 1 out]
                        n111 = call <vilib>:"Auto Power Spectrum.vi"("dt"=w342, "Signal (V)"=w339) -> ("df"=w341:dbl, "Power Spectrum (V^2 rms)"=w343:dbl[])
                      }
                      n112 = Array Size(array=w287) -> (size(s)=w306:i32[])
                      n113 = Index Array(array=w306, index=1) -> (element=w304:i32)
                      n114 = call-poly <vilib>:"Mean.vi"("X"=w293) -> ("mean"=w289:dbl)  [unwired: 1 out]
                      n115 = for {
                        N: w304 -> [_]
                        tunnel: [w331] -> w303 mode=indexing
                        i -> [w331]
                      }
                      n116 = Transpose 2D Array(2D array=w319) -> (transposed array=w320:dbl[][])
                      n117 = Multiply(x=w302, y=w303) -> (x*y=w301:dbl[])
                      n118 = expression code="X*1000"(w289) -> (w288:dbl)
                      n119 = Build Path(base path=w310, name or relative path=w313) -> (appended path=w312:path)
                      n120 = for {
                        tunnel: w320 -> [w337] mode=indexing
                        tunnel: [w336] -> w318 mode=indexing
                        n121 = call-poly <vilib>:"Mean.vi"("X"=w337) -> ("mean"=w336:dbl)  [unwired: 1 out]
                      }
                      n122 = Add(x=w300, y=w301) -> (x+y=w299:dbl[])
                      n123 = expression code="lx*1E-6"(w292) -> (w291:dbl)
                      n124 = expression code="X*1e6"(w299) -> (w298:dbl[])
                      n125 = expression code="log(x)*10"(w318) -> (w317:dbl[])
                      n126 = Build Array (concatenate)(w298, w287) -> (w297:dbl[][])
                      n127 = call-poly <vilib>:"Write To Spreadsheet File.vi"("transpose? (no:F)"=TRUE, "2D data"=w297, "file path (dialog if empty)"=w312) -> ()  [unwired: 5 in, 1 out]
                    }
                    frame #4 {
                      # "Moved back to start of local scan before moving to next element"
                      n128 = Unbundle By Name(w348) -> ("Motion Bd ID"=w349:u8)
                      n129 = expression code="x*1000"(w350) -> (w351:dbl[])
                      n130 = for {
                        N: 4 -> [_]
                        tunnel: w349 -> [w357]
                        tunnel: w351 -> [w354] mode=indexing
                        tunnel: [w353] -> w347
                        i -> [w358]
                        n131 = Increment(x=w358) -> (x+1=w355:i32)
                        n132 = call "MoveMotor.vi"("Position Mode (Absolute)"=T10."Absolute Position", "Target Position (0)"=w354, "Axis or Vector Space"=w355, "Motion Bd ID"=w357) -> ("error out"=w353:errorcluster)  [unwired: 1 in, 6 out]
                      }
                      n133 = call "FindLocation.vi"("Motion Settings"=w348, "error in (no error)"=w347) -> ("Motion Settings Out"=w346:T11)  [unwired: 1 in, 3 out]
                    }
                    frame #5 {
                      # "turn off prf"
                      n134 = Decrement(x=w362) -> (x-1=w360:i32)
                      n135 = Equal?(x=w360, y=w361) -> (x = y?=w363:bool)
                      n136 = case shown="False" w363 {
                        tunnel: w365 -> [w371 _]
                        tunnel: w364 -> [w370 _]
                        tunnel: w359 -> [w368 _]
                        frame False {
                          # "move to new location"
                          n137 = Index Array(array=w370) -> (element=w373:T3)  [unwired: 1 in]
                          n138 = call "GetScanAxis.vi"("scan pair"=w373) -> ("Axis 1"=w372:i32)  [unwired: 1 in, 2 out]
                          n139 = Unbundle By Name(w368) -> ("Motion Bd ID"=w367:u8)
                          n140 = call "MoveMotor.vi"("Position Mode (Absolute)"=T10."Relative Position", "Target Position (0)"=w371, "Axis or Vector Space"=w372, "Motion Bd ID"=w367) -> ("error out"=w369:errorcluster)  [unwired: 1 in, 6 out]
                          n141 = call "FindLocation.vi"("Motion Settings"=w368, "error in (no error)"=w369) -> ()  [unwired: 1 in, 4 out]
                        }
                        frame True {
                        }
                      }
                      n142 = call "DAQ Assistant2"("data"=bool[] [TRUE, FALSE]) -> ()  [unwired: 3 in, 16 out]
                    }
                  }
                  n143 = Build Array (concatenate)(w106, w105) -> (w104:dbl[])
                  "Current Element" <- w115
                }
                "Rms" <- w93
                "centers" <- w79
                n144 = local write "data out"(w78) -> ()
                n145 = Bundle(0, "df"=w84, w82) -> (→"Waveform Graph":cluster{i32, "df":dbl, dbl[][]})  [unwired: 1 in]
                n146 = Concatenate Strings(w91, "Pk.txt" ("string")) -> (w89:string)
                n147 = Build Path(base path=w90, name or relative path=w89) -> (appended path=w88:path)
                n148 = call-poly <vilib>:"Write To Spreadsheet File.vi"("format (%.3f)"="%.3f", "2D data"=w79, "file path (dialog if empty)"=w88) -> ()  [unwired: 5 in, 1 out]
              }
              frame #1 {
                # "Not sure what this was for"
                # "switch multiplexer"
                n149 = expression code="x*1000"(w380) -> (w381:dbl[])
                n150 = for {
                  N: 4 -> [_]
                  tunnel: w379 -> [w397]
                  tunnel: w381 -> [w394] mode=indexing
                  tunnel: [w392] -> w378
                  i -> [w393]
                  n151 = Increment(x=w393) -> (x+1=w395:i32)
                  n152 = call "MoveMotor.vi"("Position Mode (Absolute)"=T10."Absolute Position", "Target Position (0)"=w394, "Axis or Vector Space"=w395, "Motion Bd ID"=w397) -> ("error out"=w392:errorcluster)  [unwired: 1 in, 6 out]
                }
                n153 = Bundle By Name(cluster=w376, "Dig Ch"=1) -> ()  [unwired: 1 out]
                n154 = call <instrlib>:"niSwitch Disconnect All Channels.vi"("instrument handle"=w384) -> ("error out"=w385:errorcluster, "instrument handle out"=w388:refnum<k15>)  [unwired: 9 in]
                n155 = call "FindLocation.vi"("Motion Settings"=w377, "error in (no error)"=w378) -> ()  [unwired: 1 in, 4 out]
                n156 = call <instrlib>:"niSwitch Wait For Debounce.vi"("error in (no error)"=w385, "instrument handle"=w388) -> ("error out"=w386:errorcluster, "instrument handle out"=w387:refnum<k15>)  [unwired: 8 in]
                n157 = call-poly <instrlib>:"niSwitch Connect Channels.vi"("error in (no error)"=w386, "channel 2"="com0", "channel 1"="ch0", "instrument handle"=w387) -> ("error out"=w390:errorcluster, "instrument handle out"=w389:refnum<k15>)  [unwired: 6 in]
                n158 = call <instrlib>:"niSwitch Wait For Debounce.vi"("error in (no error)"=w390, "instrument handle"=w389) -> ()  [unwired: 8 in, 2 out]
              }
            }
          }
          event "Set up Digi": Value Change {
            n159 = event-data() -> ()  [unwired: 2 out]
            n160 = flat-sequence {
              tunnel: w403 -> [w404]
              tunnel: w402 -> [w411]
              tunnel: [w408] -> w401
              tunnel: w400 -> [w410]
              tunnel: [w409] -> w399
              tunnel: [w407] -> w398
              tunnel: w398 -> [w414]
              frame #0 {
                n161 = call-poly <instrlib>:"niSwitch Connect Channels.vi"("channel 2"="com0", "channel 1"="ch0", "instrument handle"=w404) -> ()  [unwired: 7 in, 2 out]
              }
              frame #1 {
                n162 = call "SetUpDigi.vi"("Digitizer Settings"=w411, "Motion Settings In"=w410, "Therapy (T)"=FALSE) -> ("Digitizer Settings Out"=w408:T5, "Motion Settings Out"=w409:T11, "Ann Array Params out"=w407:T16)  [unwired: 10 in, 4 out]
              }
              frame #2 {
                n163 = Bundle By Name(cluster=w414, "Switch T/R"=u32 0) -> ()  [unwired: 1 out]
              }
            }
          }
          event "Man Cont": Value Change {
            # "Manually move motor to desired\nlocation"
            n164 = event-data() -> ()  [unwired: 6 out]
            n165 = disable-structure shown="Enabled" {
              disable-tunnel: w416 -> [w419 w423]
              disable-tunnel: [w418 w422] -> w415
              frame Disabled {
                n166 = call "NI_controller.VI"("Motion Settings"=w419, "Initialize"=FALSE) -> ("Motion Settings Out"=w418:T11)  [unwired: 3 in, 1 out]
              }
              frame Enabled {
                n167 = call "GL_controller.VI"("Motion Settings"=w423, "Initialize"=FALSE) -> ("Motion Settings Out"=w422:T11)  [unwired: 3 in, 1 out]
              }
            }
          }
          event "home": Value Change {
            n168 = event-data() -> ()  [unwired: 6 out]
            n169 = call "NIGoHome.vi"("Board ID"=w428) -> ("error out"=w426:errorcluster)  [unwired: 2 in, 1 out]
            n170 = call "FindLocation.vi"("Motion Settings"=w425, "error in (no error)"=w426) -> ("Motion Settings Out"=w424:T11)  [unwired: 1 in, 3 out]
          }
          event "Scan": Value Change {
            n171 = event-data() -> ()  [unwired: 6 out]
            n172 = Index Array(array="data out", index (dim 0)="Scan") -> (element=w433:dbl[][])  [unwired: 2 in]
            n173 = call-poly <vilib>:"Plot Helper.vi"("z matrix"=w433) -> ("3D Plot lvclass Array out"=w432:refnum<class "3D Plot Datatype.lvclass">[])  [unwired: 5 in, 5 out]
            n174 = local write "3D Surface"(w432) -> ()
          }
        }
        n175 = Not(x="ExitSendCmd") -> (.not. x?=w46:bool)
      }
    }
  }
  n176 = local write "reset mux"(w3) -> ()
  n177 = call <instrlib>:"niSwitch Close.vi"("instrument handle"=w4) -> ()  [unwired: 10 in, 1 out]
  n178 = for {
    tunnel: w2 -> [w435] mode=indexing
    n179 = call <instrlib>:"niScope Close.vi"("instrument handle"=w435) -> ()  [unwired: 1 in, 14 out]
  }
